vi "create.vi"(8 "error in (no error)":errorcluster, 10 "configuration":T1, 11 "system.logging.provider in":refnum<class "system.logging.provider.lvclass">) -> (0 "error out":errorcluster, 3 "system.logging.provider out":refnum<class "system.logging.provider.lvclass">)   [LabVIEW 2021, in "system.logging.provider.lvclass"]
uses:
  system.logging.provider.lvclass
  system.logging/configuration.ctl
  system.logging/severity.ctl
  system.logging.provider.lvclass/system.logging.provider.ctl
  system.logging/system.logging.lvclass
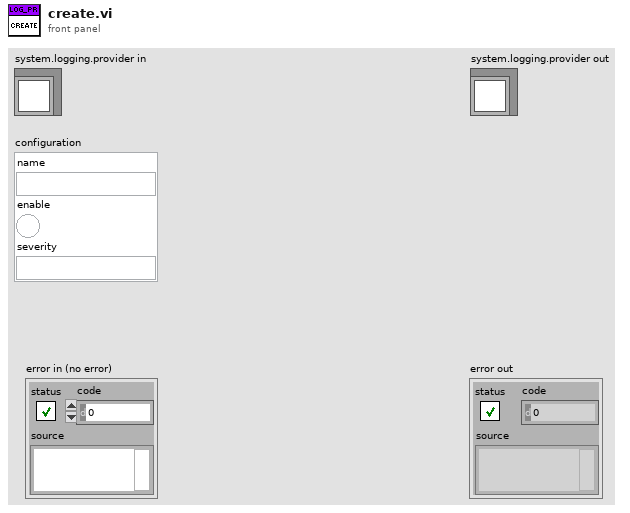
[diagram p1: front panel]
types:
  T1 = typedef "system.logging.lvclass/configuration.ctl" = cluster{"name":string, "enable":bool, "severity":string}
  T2 = typedef "system.logging.lvclass/severity.ctl" = enum8{"trace", "debug", "info", "warning", "error"}
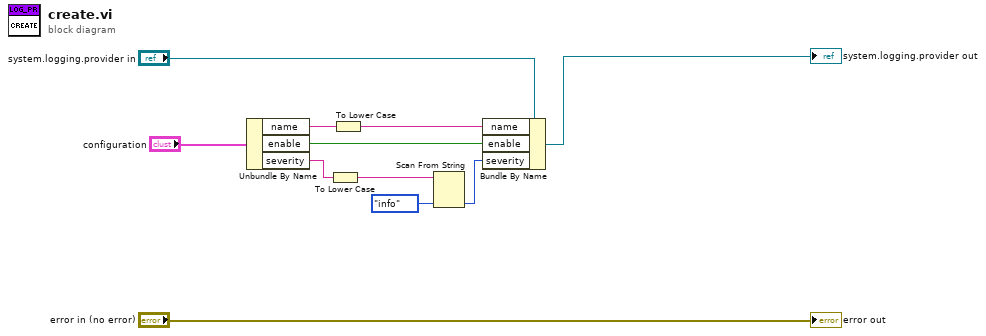
[diagram p0: block diagram]
diagram:
  n1 = Unbundle By Name("configuration") -> ("name"=w5:string, "enable"=w9:bool, "severity"=w6:string)
  n2 = To Lower Case(string=w6) -> (all lower case string=w3:string)
  n3 = To Lower Case(string=w5) -> (all lower case string=w4:string)
  n4 = Scan From String(input string=w3, default 1=severity."info" ("severity")) -> (output 1=w7:T2)  [unwired: 3 in, 3 out]
  n5 = Bundle By Name(cluster="system.logging.provider in", "name"=w4, "enable"=w9, "severity"=w7) -> (→"system.logging.provider out":refnum<class "system.logging.provider.lvclass">)
  "error out" <- "error in (no error)"
